vi "Main.vi"() -> ()   [LabVIEW 2018]
uses:
  TypeDefs/cntlRefs.ctl
  NistPluggableModules/BusClass/Bus.lvclass/Bus.ctl
  LV_Config_class/Typedefs/eLogLvl.ctl
  LV_Config_class/Config.lvclass/Config.ctl
  NistPluggableModules/BusClass/Accessors/Read Test.vi
  LV_Config_class/Accessors/Read ConfigFilePath.vi
  NistPluggableModules/BusClass/Accessors/Read BusNumber.vi
  <vilib>/Utility/error.llb/Error Cluster From Error Code.vi
  <vilib>/ErrorRing/Error Ring.xnode
  NistPluggableModules/TestClass/Test.lvclass
  Queue/Queue.lvlib
  <userlib>/NIST/NISTErrorLib/NISTErrorLib.lvlib
  LV_Config_class/Config.lvclass
  LV_Ini/Ini_lib.lvlib
  <vilib>/Utility/config.llb/NI_LVConfig.lvlib
  NistPluggableModules/BusClass/Bus.lvclass
  NistPluggableModules/Visualization/Visualization.lvlib
panel:
  in  "Blank Button":bool
  in  "ConfigurationList":bool[](array[boolean])
  in  "InstrumentList":u16[](array[ring]) items=["Agilent IVI FGen", "IVI Dual FGens"]
  in  "btnNHRDCPref":bool
  in  "btnNHRGSPref":bool
  in  "btnPPSPref":bool
  in  "btnChromaDCPref":bool
  in  "rngNHRDC":u16(ring) caption="NHR DC Power" items=["Agilent IVI FGen", "IVI Dual FGens"]
  in  "rngNHRG":u16(ring) caption="NHR GridSimulator" items=["Agilent IVI FGen", "IVI Dual FGens"]
  in  "rngPPS":u16(ring) caption="PPS" items=["AcPwrBase", "Chroma", "ChromaDCLoad", "NHRDCPower", "PPS"]
  in  "rngChromaDC":u16(ring) caption="ChromaDC" items=["Agilent IVI FGen", "IVI Dual FGens"]
  in  "btnChromaACPref":bool
  in  "rngChromaAC":u16(ring) caption="ChromaAC" items=["AcPwrBase", "Chroma", "ChromaDCLoad", "NHRDCPower", "PPS"]
  in  "ModuleList":string[](array[string])=["AcPwr.Chroma"]
  in  "btnRunOne":bool
  in  "btnVisualization":bool caption="Visualization"
  in  "btnHide":bool caption="Hide Modules"
  in  "btnSettings":bool
  in  "btnStop":bool
  in  "btnFGenPref":bool
  in  "rngFGen":u16(ring) caption="Function Generator" items=["Agilent IVI FGen", "IVI Dual FGens"]
  in  "rngDigitizer":u16(ring) caption="Digitizer" items=["IVI Digitizer", "Analyse Waveforms", "Debug", "Ni DaqMx Digitizer", "PMU Cal", "(obsolete)", "Simulation"]
  in  "btnDigitizerPref":bool
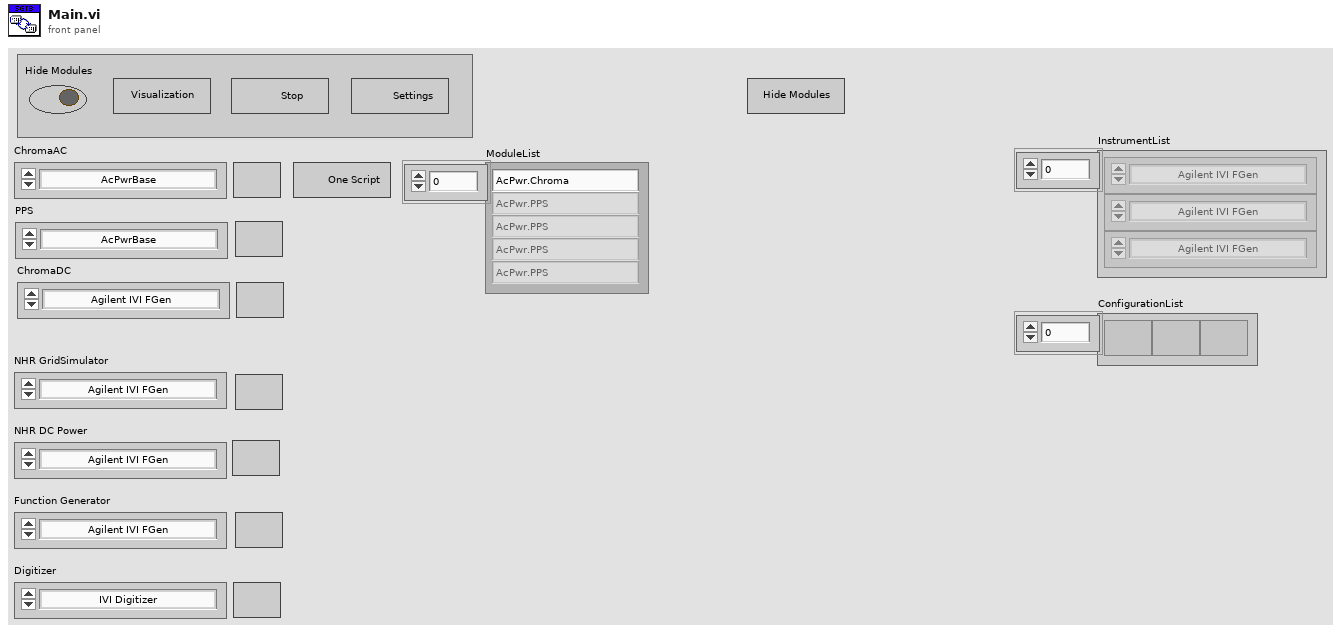
[diagram p1: front panel]
types:
  T1 = typedef "cntlRefs.ctl" = cluster{"rngFGen":refnum<vi>, "rngDigitizer":refnum<vi>, "btnHide":refnum<vi>, "rngChromaAC":refnum<vi>, "rngChromaDC":refnum<vi>, "rngPPS":refnum<vi>, "rngNHRG":refnum<vi>, "rngNHRDC":refnum<vi>}
  T2 = typedef "clUserEvents.ctl" = cluster{"StopEvent":refnum<user-event>, "RefreshUserEvents":refnum<user-event>}
  T3 = typedef "FgenModule.lvlib/clBroadcastEvents.ctl" = cluster{"DidInit":refnum<user-event>, "StatusUpdate":refnum<user-event>, "ErrorReport":refnum<user-event>, "DidStop":refnum<user-event>, "PathToINI":refnum<user-event>, "Channels":refnum<user-event>, "Function":refnum<user-event>, "Waveforms":refnum<user-event>, "Triggers":refnum<user-event>, "FunctionParams":refnum<user-event>}
  T4 = typedef "ScopeModule.lvlib/clBroadcastEvents.ctl" = cluster{"DidInit":refnum<user-event>, "StatusUpdate":refnum<user-event>, "ErrorReport":refnum<user-event>, "DidStop":refnum<user-event>, "PathToINI":refnum<user-event>, "Handle":refnum<user-event>, "Model":refnum<user-event>, "Channels":refnum<user-event>, "Acquisition":refnum<user-event>, "Trigger":refnum<user-event>, "ExtAcquisition":refnum<user-event>, "Waveform":refnum<user-event>}
  T5 = typedef "AcPwrModule.lvlib/clBroadcastEvents.ctl" = cluster{"DidInit":refnum<user-event>, "StatusUpdate":refnum<user-event>, "ErrorReport":refnum<user-event>, "DidStop":refnum<user-event>, "PathToINI":refnum<user-event>, "Measurements":refnum<user-event>, "LoadConfigFile":refnum<user-event>, "GetSettings":refnum<user-event>, "SetSettings":refnum<user-event>, "GetType&ID":refnum<user-event>}
  T6 = typedef "Config_class.lvlib/Config.lvclass/eLogLvl.ctl" = enum16{"Normal", "Verbose", "None"}
  T7 = typedef "NI_LVConfig.lvlib/Config Data RefNum.ctl" = refnum<k1>
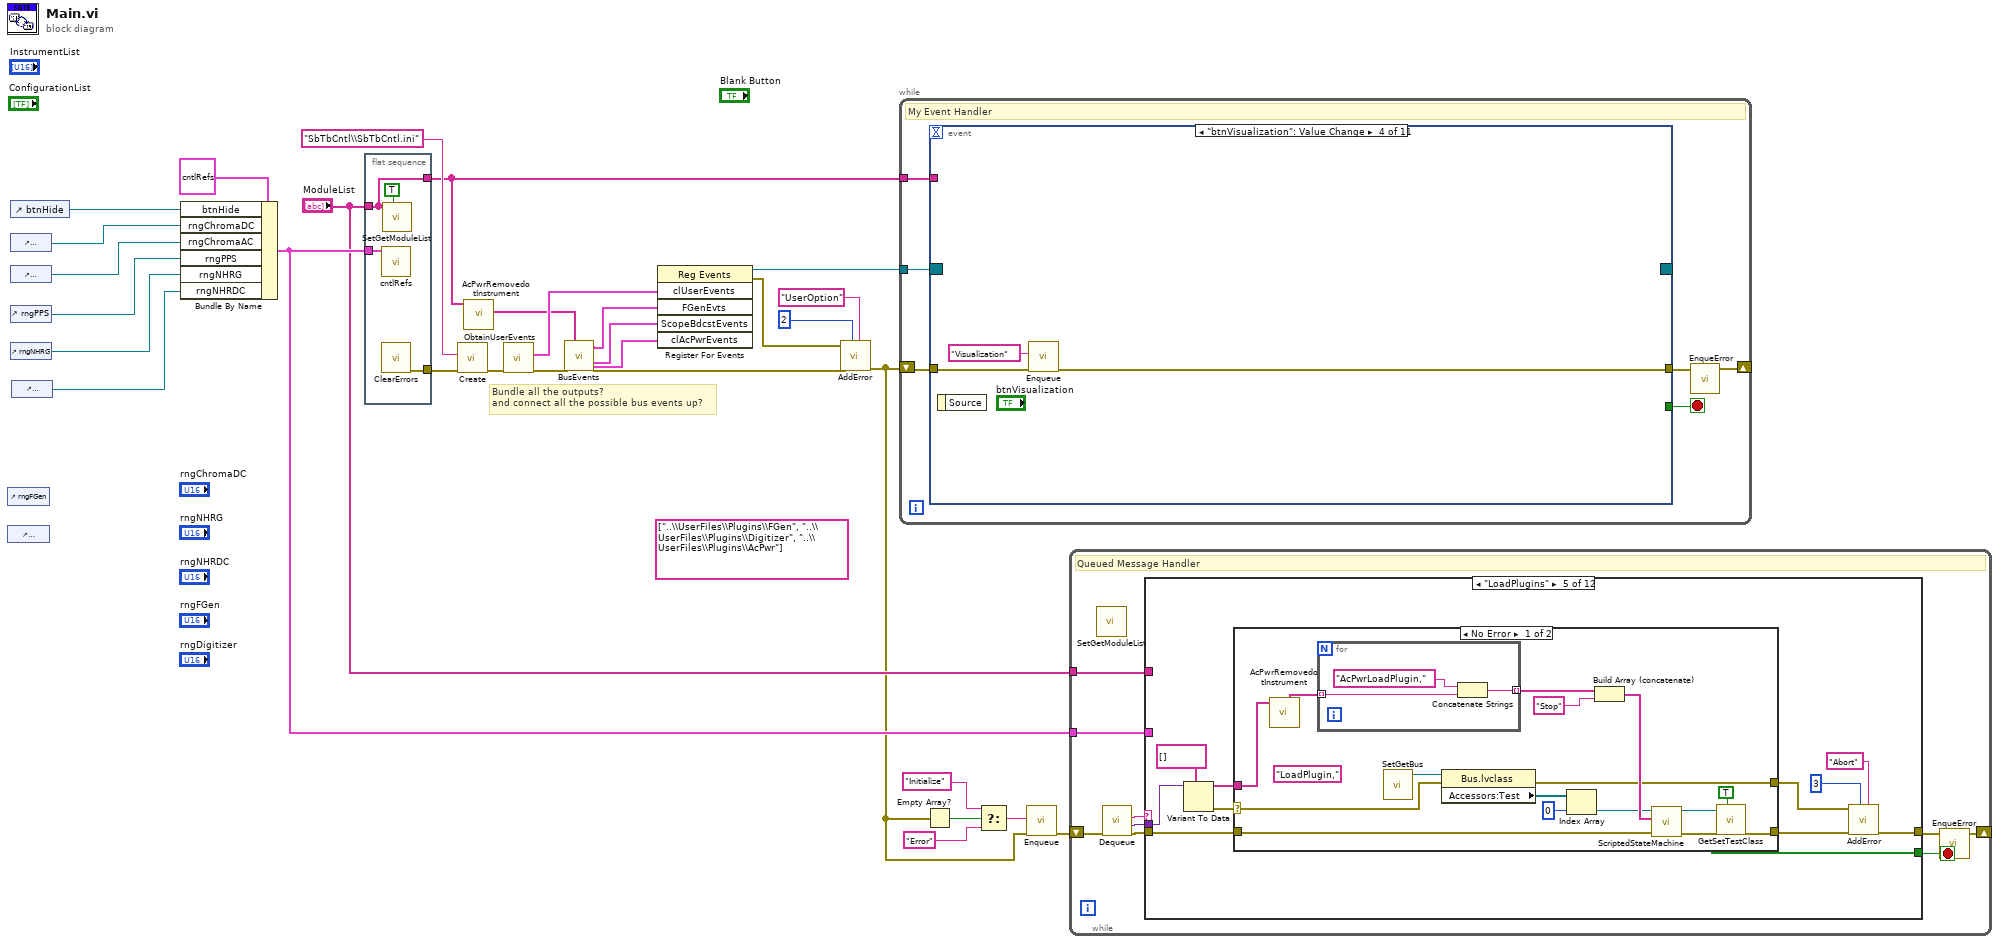
[diagram p0: block diagram]
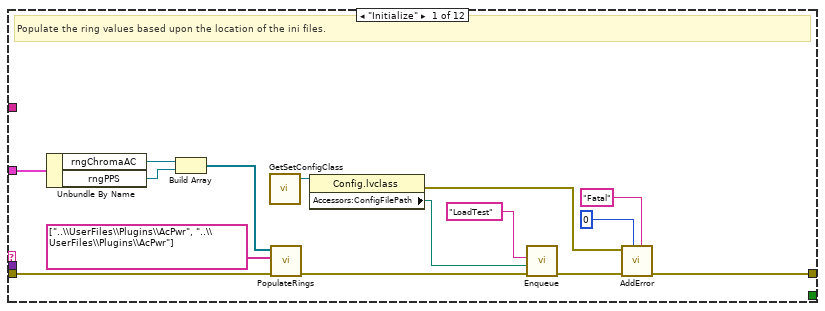
[diagram p2: hidden frame]
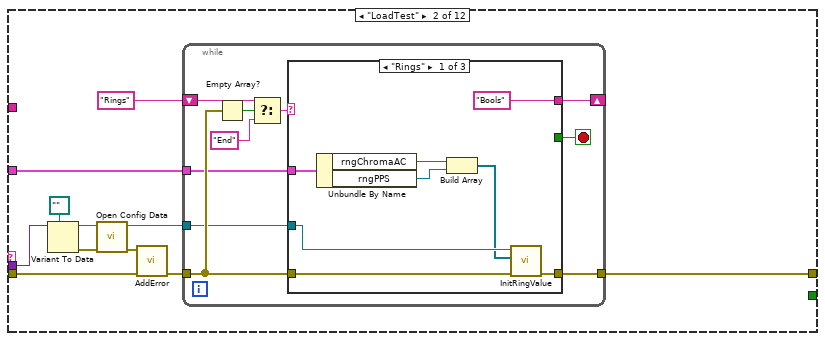
[diagram p3: hidden frame]
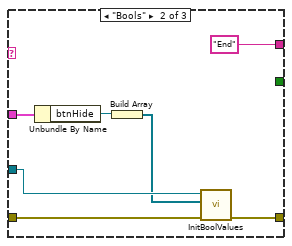
[diagram p4: hidden frame]
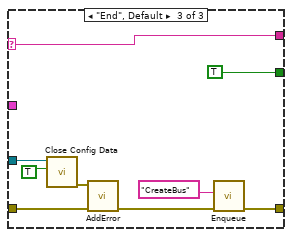
[diagram p5: hidden frame]
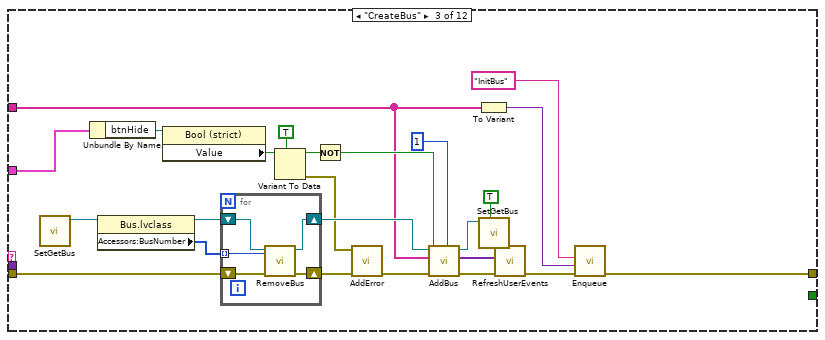
[diagram p6: hidden frame]
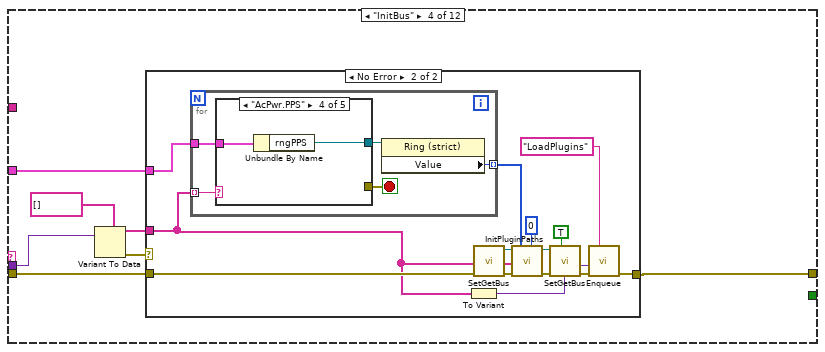
[diagram p7: hidden frame]
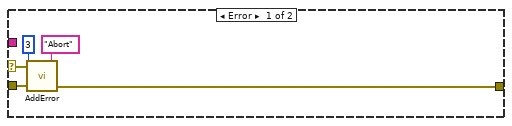
[diagram p8: hidden frame]
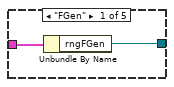
[diagram p9: hidden frame]
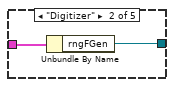
[diagram p10: hidden frame]
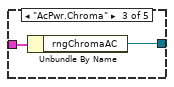
[diagram p11: hidden frame]
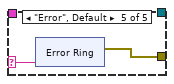
[diagram p12: hidden frame]
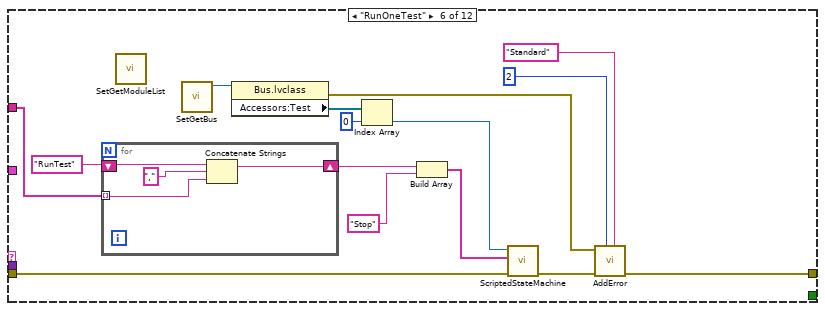
[diagram p14: hidden frame]
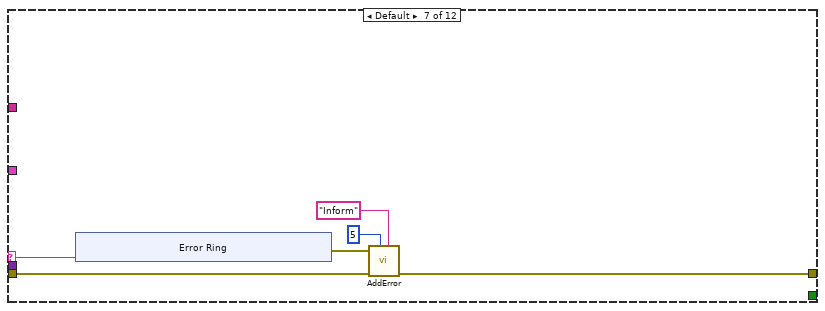
[diagram p15: hidden frame]
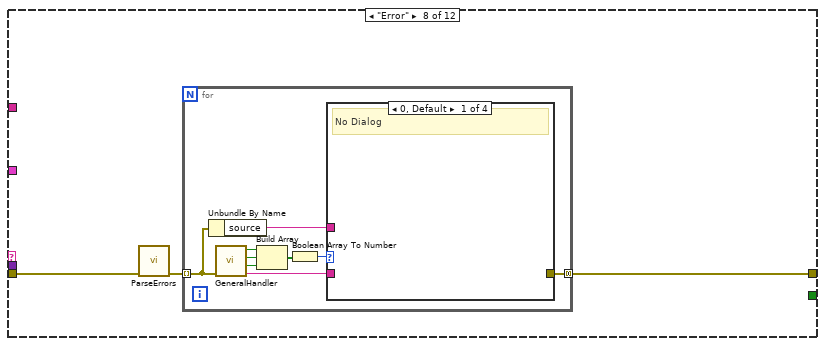
[diagram p16: hidden frame]
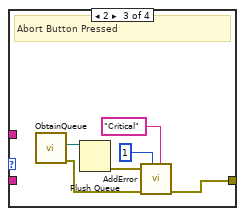
[diagram p19: hidden frame]
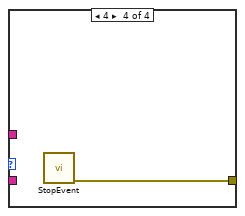
[diagram p20: hidden frame]
diagram:
  (unwired) string[] ["..\\UserFiles\\Plugins\\FGen", "..\\UserFiles\\Plugins\\Digitizer", "..\\UserFiles\\Plugins\\AcPwr"] ("RelativePathToIniArray")
  # "Bundle all the outputs? \nand connect all the possible bus events up?"
  n1 = control-ref of="rngFGen"() -> ()  [unwired: 1 out]
  n2 = control-ref of="rngDigitizer"() -> ()  [unwired: 1 out]
  n3 = control-ref of="btnHide"() -> (w15:refnum<vi>)
  n4 = control-ref of="rngChromaDC"() -> (w14:refnum<vi>)
  n5 = control-ref of="rngChromaAC"() -> (w13:refnum<vi>)
  n6 = control-ref of="rngPPS"() -> (w12:refnum<vi>)
  n7 = control-ref of="rngNHRG"() -> (w11:refnum<vi>)
  n8 = control-ref of="rngNHRDC"() -> (w10:refnum<vi>)
  n9 = Bundle By Name(cluster=T1 {"rngFGen"=refnum, "rngDigitizer"=refnum, "btnHide"=refnum, "rngChromaAC"=refnum, "rngChromaDC"=refnum, "rngPPS"=refnum, "rngNHRG"=refnum, "rngNHRDC"=refnum} ("cntlRefs"), "btnHide"=w15, "rngChromaDC"=w14, "rngChromaAC"=w13, "rngPPS"=w12, "rngNHRG"=w11, "rngNHRDC"=w10) -> (w9:T1)
  n10 = flat-sequence {
    tunnel: [w34] -> w19
    tunnel: w9 -> [w33]
    tunnel: "ModuleList" -> [w31]
    tunnel: [w31] -> w2
    frame #0 {
      n11 = call "cntlRefs.vi"("cntlRefs"=w33) -> ()  [unwired: 10 in, 1 out]
      n12 = call <userlib>:"ClearErrors.vi"() -> ("ErrorArray"=w34:errorcluster[])  [unwired: 11 in]
      n13 = call "SetGetModuleList.vi"("Set? (f)"=TRUE, "ModuleList"=w31) -> ()  [unwired: 9 in, 1 out]
    }
  }
  n14 = call "Create.vi"("ErrorArray"=w19, "name or relative path"="SbTbCntl\\SbTbCntl.ini") -> ("ErrorArray"=w20:errorcluster[])  [unwired: 8 in, 1 out]
  n15 = call "AcPwrRemovedotInstrument.vi"("ModuleList"=w2) -> ("BeforeMatch-RedundantEntries"=w1:string[])  [unwired: 8 in, 2 out]
  n16 = call "ObtainUserEvents.vi"("ErrorArray"=w20) -> ("ErrorArray"=w21:errorcluster[], "clUserEvents"=w29:T2)  [unwired: 9 in]
  n17 = call "BusEvents.vi"("Error in"=w21, "ModuleList"=w1) -> ("FGenEvts"=w16:T3, "ScopeBdcstEvents"=w18:T4, "clAcPwrEvents"=w17:T5, "Error out"=w6:errorcluster[])  [unwired: 18 in, 4 out]
  n18 = register-events(w29, w16, w18, w17) -> (reference out=w30:refnum<event-registration>, error out=w5:errorcluster)  [unwired: 2 in]
  n19 = call <userlib>:"AddError.vi"("Severity"="UserOption", "Priority"=u8 2, "ErrorArray"=w6, "error in (no error)"=w5) -> ("ErrorArray"=w3:errorcluster[])  [unwired: 6 in, 1 out]
  n20 = while {
    tunnel: w30 -> [w40]
    shift-right: [w37] -> _
    shift-left: w3 -> [w39]
    tunnel: w2 -> [w35]
    stop <- w36 stop-if-true
    # "My Event Handler"
    n21 = event shown="[3] \"btnVisualization\": Value Change" {
      selector: w40 -> [_ _ _ _ _ _ _ _ _ w210 _]
      dyn-events: [_ _ _ _ _ _ _ _ _ w211 _] -> _
      timeout: _ -> [_ _ _ _ _ _ _ _ _ _ _]
      tunnel: w39 -> [w42 w47 w61 w70 w73 w76 w123 w173 w187 w201 w214]
      tunnel: [w41 w46 w62 w69 w72 w77 w124 w164 w183 w199 w213] -> w38
      tunnel: [_ "btnStop" _ _ _ _ _ _ _ _ TRUE] -> w36
      tunnel: w35 -> [_ _ w49 _ _ _ _ _ _ w204 _]
      event "btnSettings": Value Change {
        n22 = event-data() -> ()  [unwired: 1 in, 1 out]
        n23 = call "Settings.vi"("ErrorArray"=w42) -> ("ErrorArray"=w41:errorcluster[])  [unwired: 10 in]
      }
      event "btnStop": Value Change {
        # "Stops the Framework and sends a message to the queued message handler to stop."
        n24 = event-data() -> ()  [unwired: 1 in, 1 out]
        n25 = call "Enqueue.vi"("Priority (F)"=TRUE, "ErrorArray"=w47, "Message"="Stop") -> ("ErrorArray"=w46:errorcluster[])  [unwired: 8 in]
      }
      event "btnHide": Value Change {
        # "Displays the modules need to fix this for AcPwr"
        n26 = event-data() -> ("NewVal"=w57:bool)  [unwired: 1 in]
        n27 = call "AcPwrRemovedotInstrument.vi"("ModuleList"=w49) -> ("Before Match"=w48:string[])  [unwired: 8 in, 2 out]
        n28 = call "SetGetBus.vi"() -> ("Bus.lvclass"=w60:refnum<class "Bus.lvclass">)  [unwired: 11 in]
        n29 = call "SetGetModuleList.vi"() -> ()  [unwired: 11 in, 1 out]
        n30 = property class="Bus.lvclass"(reference=w60) -> ("Accessors:Test"=w59:refnum<class "Test.lvclass">[])  [unwired: 1 in, 2 out]
        n31 = Select(t="false", s=w57, f="true") -> (s? t:f=w50:string)
        n32 = for {
          tunnel: [w67] -> w51 mode=indexing
          tunnel: w48 -> [w65] mode=indexing
          tunnel: w50 -> [w63]
          n33 = Concatenate Strings("AcPwrHideModule,", w65, ",", w63) -> (w67:string)
        }
        n34 = Index Array(array=w59, index=0) -> (element=w58:refnum<class "Test.lvclass">)
        n35 = Build Array (concatenate)(w51, "Stop") -> (w53:string[])
        n36 = call "ScriptedStateMachine.vi"("ErrorArray"=w61, "script"=w53, "Test.lvclass"=w58) -> ("ErrorArray"=w62:errorcluster[])  [unwired: 6 in, 2 out]
      }
      event "btnVisualization": Value Change {
        n37 = event-data() -> ()  [unwired: 1 in, 1 out]
        n38 = call "Enqueue.vi"("ErrorArray"=w70, "Message"="Visualization") -> ("ErrorArray"=w69:errorcluster[])  [unwired: 9 in]
      }
      event "btnRunOne": Value Change {
        # "Runs a single test?"
        n39 = event-data() -> ()  [unwired: 1 in, 1 out]
        n40 = call "Enqueue.vi"("ErrorArray"=w73, "Message"="RunOneTest") -> ("ErrorArray"=w72:errorcluster[])  [unwired: 9 in]
      }
      event "btnFGenPref", "btnDigitizerPref", "btnChromaACPref", "btnChromaDCPref", "btnPPSPref", "btnNHRGSPref", "btnNHRDCPref": Value Change {
        # "Sends a command to open up the preferences dialog. This case needs some more work but is currently runnable"
        n41 = event-data() -> ("CtlRef"=w80:refnum<vi>)  [unwired: 1 in]
        n42 = property class="Bool (strict)"(reference=w80) -> (error out=w74:errorcluster, "Label.Text"=w79:string)  [unwired: 1 in, 1 out]
        n43 = case shown="\"btnPPSPref\"" w79 {
          selector: w79 -> [_ _ _ _ w108]
          tunnel: ["Digitizer" "FGen" "Chroma" "PPS" "Error"] -> w78
          tunnel: [w98 w100 w102 w104 w107] -> w75
          tunnel: w74 -> [w98 w100 w102 w104 _]
          frame "btnDigitizerPref" {
          }
          frame "btnFGenPref" {
          }
          frame "btnChromaACPref" {
          }
          frame "btnPPSPref" {
          }
          frame Default {
            n44 = xnode "Error Ring"("parameter 0"=w108) -> ("error out"=w107:errorcluster)
          }
        }
        n45 = case shown="No Error" w75 {
          selector: w75 -> [w82 w95]
          tunnel: w78 -> [w83 _]
          tunnel: [w91 w97] -> w77
          tunnel: w76 -> [w90 w96]
          frame No Error {
            (unwired) "PrefDlgRequest," ("string")
            n46 = call "SetGetBus.vi"() -> ("Bus.lvclass"=w87:refnum<class "Bus.lvclass">)  [unwired: 11 in]
            n47 = property class="Bus.lvclass"(reference=w87, error in=w82) -> ("Accessors:Test"=w86:refnum<class "Test.lvclass">[])  [unwired: 2 out]
            n48 = Concatenate Strings("AcPwrPrefDlg," ("string"), w83) -> (w92:string)
            n49 = Build Array(w92, "Stop" ("element")) -> (w89:string[])
            n50 = Index Array(array=w86, index=0) -> (element=w85:refnum<class "Test.lvclass">)
            n51 = call "ScriptedStateMachine.vi"("ErrorArray"=w90, "script"=w89, "Test.lvclass"=w85) -> ("ErrorArray"=w91:errorcluster[])  [unwired: 6 in, 2 out]
          }
          frame Error {
            n52 = call <userlib>:"AddError.vi"("Severity"="Abort", "Priority"=u8 0, "ErrorArray"=w96, "error in (no error)"=w95) -> ("ErrorArray"=w97:errorcluster[])  [unwired: 6 in, 1 out]
          }
        }
      }
      event "rngFGen", "rngDigitizer", "rngChromaAC", "rngChromaDC", "rngPPS", "rngNHRG", "rngNHRDC": Value Change {
        # "Also needs some work"
        n53 = event-data() -> ("CtlRef"=w128:refnum<vi>)  [unwired: 1 in]
        n54 = call "SetGetBus.vi"() -> ("Bus.lvclass"=w122:refnum<class "Bus.lvclass">)  [unwired: 11 in]
        n55 = property class="Bus.lvclass"(reference=w122) -> (error out=w116:errorcluster, "Accessors:Test"=w119:refnum<class "Test.lvclass">[])  [unwired: 1 in, 1 out]
        n56 = property class="Ring (strict)"(reference=w128, error in=w116) -> (error out=w117:errorcluster, "Label.Text"=w127:string, "Value"=w121:u16)  [unwired: 1 out]
        n57 = Index Array(array=w119, index=0) -> (element=w118:refnum<class "Test.lvclass">)
        n58 = case shown="\"ChromaAC\"" w127 {
          selector: w127 -> [w146 _ _ _ _]
          tunnel: [_ "Digitizer" "FGen" "Chroma" "PPS"] -> w126
          tunnel: [w145 w152 w154 w156 w158] -> w125
          tunnel: w117 -> [_ w152 w154 w156 w158]
          frame Default {
            n59 = xnode ("Error Ring")("parameter 0"=w146) -> ("error out"=w145:errorcluster)
          }
          frame "rngDigitizer" {
          }
          frame "rngFGen" {
          }
          frame "ChromaAC" {
          }
          frame "PPS" {
          }
        }
        n60 = case shown="No Error" w125 {
          selector: w125 -> [_ w142]
          tunnel: w126 -> [w132 _]
          tunnel: [w138 w144] -> w124
          tunnel: w123 -> [w134 w143]
          tunnel: w121 -> [w133 _]
          tunnel: w118 -> [w131 _]
          frame No Error {
            (unwired) "LoadPlugin," ("string")
            n61 = call "UpdatePluginIndex.vi"("Error"=w134, "Index"=w133, "PluginName"=w132, "Test"=w131) -> ("Error"=w135:errorcluster[], "Test"=w130:refnum<class "Test.lvclass">)  [unwired: 6 in]
            n62 = Concatenate Strings("AcPwrLoadPlugin," ("string"), w132) -> (w139:string)
            n63 = Build Array(w139, "Stop") -> (w137:string[])
            n64 = call "ScriptedStateMachine.vi"("ErrorArray"=w135, "script"=w137, "Test.lvclass"=w130) -> ("ErrorArray"=w138:errorcluster[])  [unwired: 6 in, 2 out]
          }
          frame Error {
            n65 = call <userlib>:"AddError.vi"("Severity"="Abort", "Priority"=u8 3, "ErrorArray"=w143, "error in (no error)"=w142) -> ("ErrorArray"=w144:errorcluster[])  [unwired: 6 in, 1 out]
          }
        }
      }
      event User Event {
        # "Logs any error that occurs in each module"
        n66 = event-data() -> ("ModuleID"=w172:i32, "Data"=w177:variant)  [unwired: 1 in]
        n67 = Get Date/Time In Seconds() -> (seconds since 1Jan1904=w176:timestamp)
        n68 = Get Date/Time String(date format (0)=enum16{"short", "long", "abbreviated"}."short", seconds (now)=w176, want seconds? (F)=TRUE) -> (time string=w175:string)  [unwired: 1 out]
        n69 = Variant To Data(type=errorcluster {"status"=FALSE, "code"=0, "source"=""} ("error in (no error)"), Variant=w177) -> (data=w167:errorcluster, error out=w169:errorcluster)  [unwired: 1 in]
        n70 = Unbundle By Name(w167) -> ("source"=w166:string)
        n71 = Merge Errors(w167, w169) -> (w161:errorcluster)
        n72 = Format Into String(format string="%s: Module %d: %s \\r", error in=w161, w175, w172, w166) -> (resulting string=w162:string, error out=w160:errorcluster)  [unwired: 1 in]
        n73 = call <userlib>:"AddError.vi"("Severity"="Standard", "Priority"=u8 2, "ErrorArray"=w173, "error in (no error)"=w160) -> ("ErrorArray"=w165:errorcluster[])  [unwired: 6 in, 1 out]
        n74 = call "LogMessage.vi"("eLogLvl"=eLogLvl."Normal" ("LogLevel"), "Error"=w165, "LogMessage"=w162) -> ("Error"=w164:errorcluster[])  [unwired: 8 in]
      }
      event User Event {
        # "Logs and Status Update from the modules"
        n75 = event-data() -> ("Data"=w193:variant)  [unwired: 1 in]
        n76 = Get Date/Time In Seconds() -> (seconds since 1Jan1904=w194:timestamp)
        n77 = Variant To Data(type="", Variant=w193) -> (data=w190:string, error out=w192:errorcluster)  [unwired: 1 in]
        n78 = Get Date/Time String(date format (0)=enum16{"short", "long", "abbreviated"}."short", seconds (now)=w194, want seconds? (F)=TRUE) -> (time string=w191:string)  [unwired: 1 out]
        n79 = Format Into String(format string="%s: %s \\r", error in=w192, w191, w190) -> (resulting string=w180:string, error out=w186:errorcluster)  [unwired: 1 in]
        n80 = call <userlib>:"AddError.vi"("Severity"="Inform", "Priority"=u8 4, "ErrorArray"=w187, "error in (no error)"=w186) -> ("ErrorArray"=w182:errorcluster[])  [unwired: 6 in, 1 out]
        n81 = call "LogMessage.vi"("eLogLvl"=eLogLvl."Normal", "Error"=w182, "LogMessage"=w180) -> ("Error"=w183:errorcluster[])  [unwired: 8 in]
      }
      event User Event {
        # "Connect all the bus events on the external call and internal call?"
        n82 = event-data() -> ("Data"=w212:variant)  [unwired: 1 in]
        n83 = Variant To Data(type=variant[] [] ("UsrEvents"), Variant=w212) -> (data=w209:variant[], error out=w203:errorcluster)  [unwired: 1 in]
        n84 = call "SetGetModuleList.vi"() -> ()  [unwired: 11 in, 1 out]
        n85 = call "BusEvents.vi"("EventArray"=w209, "Error in"=w201, "ModuleList"=w204) -> ("FGenEvts"=w205:T3, "ScopeBdcstEvents"=w206:T4, "clAcPwrEvents"=w207:T5, "Error out"=w200:errorcluster[])  [unwired: 17 in, 4 out]
        n86 = register-events(reference=w210, error in=w203, w205, w206, w207) -> (reference out=w211:refnum<event-registration>, error out=w202:errorcluster)  [unwired: 1 in]
        n87 = call <userlib>:"AddError.vi"("Severity"="Fatal", "Priority"=u8 0, "ErrorArray"=w200, "error in (no error)"=w202) -> ("ErrorArray"=w199:errorcluster[])  [unwired: 6 in, 1 out]
      }
      event User Event {
        # "Queued Message Handler stops for any reason this top loop needs to also stop or an external stop call."
        n88 = event-data() -> ()  [unwired: 1 in, 1 out]
        n89 = call "Enqueue.vi"("Priority (F)"=TRUE, "ErrorArray"=w214, "Message"="Stop") -> ("ErrorArray"=w213:errorcluster[])  [unwired: 8 in]
      }
    }
    n90 = call "EnqueError.vi"("ErrorArrayIn"=w38) -> ("ErrorArrayOut"=w37:errorcluster[])  [unwired: 10 in]
  }
  n91 = Empty Array?(array=w3) -> (empty?=w25:bool)
  n92 = Select(t="Initialize" ("Message"), s=w25, f="Error") -> (s? t:f=w22:string)
  n93 = call "Enqueue.vi"("ErrorArray"=w3, "Message"=w22) -> ("ErrorArray"=w28:errorcluster[])  [unwired: 9 in]
  n94 = while {
    shift-right: [w223] -> _
    shift-left: w28 -> [w226]
    tunnel: w9 -> [w219]
    tunnel: "ModuleList" -> [w218]
    stop <- w221 stop-if-true
    # "Queued Message Handler"
    n95 = call "SetGetModuleList.vi"() -> ()  [unwired: 11 in, 1 out]
    n96 = call "Dequeue.vi"("ErrorArray"=w226) -> ("ErrorArray"=w222:errorcluster[], "Message Data"=w220:variant, "Message"=w225:string)  [unwired: 8 in]
    n97 = case shown="\"LoadPlugins\"" w225 {
      selector: w225 -> [_ _ _ _ _ _ w414 _ _ _ _ _]
      tunnel: [w227 w251 w300 w320 w362 w391 w413 w423 w443 w447 w466 w502] -> w224
      tunnel: w222 -> [w241 w248 w310 w321 w368 w401 w412 w422 w444 w446 w460 w506]
      tunnel: [_ _ _ _ _ _ _ _ _ _ _ TRUE] -> w221
      tunnel: w220 -> [_ w244 _ w322 w367 _ _ _ _ _ w464 _]
      tunnel: w219 -> [w234 w242 w288 w316 _ _ _ _ _ _ w456 _]
      tunnel: w218 -> [_ _ w287 _ _ w390 _ _ _ _ _ _]
      frame "Initialize" {
        # "Populate the ring values based upon the location of the ini files."
        n98 = Unbundle By Name(w234) -> ("rngChromaAC"=w233:refnum<vi>, "rngPPS"=w232:refnum<vi>)
        n99 = Build Array(w233, w232) -> (w235:refnum<vi>[])
        n100 = call "GetSetConfigClass.vi"() -> ("Ref out"=w237:refnum<class "Config.lvclass">)  [unwired: 11 in]
        n101 = call "PopulateRings.vi"("ErrorArray In"=w241, "RelativePathToIniArray"=string[] ["..\\UserFiles\\Plugins\\AcPwr", "..\\UserFiles\\Plugins\\AcPwr"], "RingRefArray"=w235) -> ("ErrorArray Out"=w239:errorcluster[])  [unwired: 7 in, 1 out]
        n102 = property class="Config.lvclass"(reference=w237) -> (error out=w229:errorcluster, "Accessors:ConfigFilePath"=w236:path)  [unwired: 1 in, 1 out]
        n103 = call "Enqueue.vi"("ErrorArray"=w239, "Message Data"=w236, "Message"="LoadTest") -> ("ErrorArray"=w228:errorcluster[])  [unwired: 8 in]
        n104 = call <userlib>:"AddError.vi"("Severity"="Fatal", "Priority"=u8 0, "ErrorArray"=w228, "error in (no error)"=w229) -> ("ErrorArray"=w227:errorcluster[])  [unwired: 6 in, 1 out]
      }
      frame "LoadTest" {
        n105 = Variant To Data(type=path "", Variant=w244) -> (data=w245:path, error out=w250:errorcluster)  [unwired: 1 in]
        n106 = call <vilib>:"Open Config Data.vi"("error in (no error)"=w250, "configuration file path"=w245) -> ("error out"=w247:errorcluster, "refnum"=w243:T7)  [unwired: 7 in, 1 out]
        n107 = call <userlib>:"AddError.vi"("ErrorArray"=w248, "error in (no error)"=w247) -> ("ErrorArray"=w249:errorcluster[])  [unwired: 8 in, 1 out]
        n108 = while {
          shift-right: [w262] -> _
          shift-left: "Rings" -> [w255]
          tunnel: w249 -> [w257]
          tunnel: [w259] -> w251
          tunnel: w243 -> [w254]
          tunnel: w242 -> [w253]
          stop <- w258 stop-if-true
          n109 = Empty Array?(array=w257) -> (empty?=w256:bool)
          n110 = Select(t=w255, s=w256, f="End") -> (s? t:f=w261:string)
          n111 = case shown="\"Rings\"" w261 {
            selector: w261 -> [_ _ w286]
            tunnel: ["Bools" "End" w286] -> w262
            tunnel: w257 -> [w268 w275 w281]
            tunnel: [w269 w276 w280] -> w259
            tunnel: [_ _ TRUE] -> w258
            tunnel: w254 -> [w267 w273 w284]
            tunnel: w253 -> [w265 w272 _]
            frame "Rings" {
              n112 = Unbundle By Name(w265) -> ("rngChromaAC"=w266:refnum<vi>, "rngPPS"=w264:refnum<vi>)
              n113 = Build Array(w266, w264) -> (w263:refnum<vi>[])
              n114 = call "InitRingValue.vi"("ErrorArray In"=w268, "RingRefArray"=w263, "IniFileRef"=w267) -> ("ErrorArray Out"=w269:errorcluster[])  [unwired: 6 in, 2 out]
            }
            frame "Bools" {
              n115 = Unbundle By Name(w272) -> ("btnHide"=w274:refnum<vi>)
              n116 = Build Array(w274) -> (w271:refnum<vi>[])
              n117 = call "InitBoolValues.vi"("ErrorArray in"=w275, "BoolRefArray"=w271, "IniFileRef in"=w273) -> ("ErrorArray Out"=w276:errorcluster[])  [unwired: 7 in, 1 out]
            }
            frame "End", Default {
              n118 = call <vilib>:"Close Config Data.vi"("write file if changed (T)"=TRUE, "refnum"=w284) -> ("error out"=w282:errorcluster)  [unwired: 8 in, 1 out]
              n119 = call <userlib>:"AddError.vi"("ErrorArray"=w281, "error in (no error)"=w282) -> ("ErrorArray"=w279:errorcluster[])  [unwired: 8 in, 1 out]
              n120 = call "Enqueue.vi"("ErrorArray"=w279, "Message"="CreateBus") -> ("ErrorArray"=w280:errorcluster[])  [unwired: 9 in]
            }
          }
        }
      }
      frame "CreateBus" {
        n121 = call "SetGetBus.vi"() -> ("Bus.lvclass"=w306:refnum<class "Bus.lvclass">)  [unwired: 11 in]
        n122 = Unbundle By Name(w288) -> ("btnHide"=w289:refnum<vi>)
        n123 = property class="Bus.lvclass"(reference=w306) -> (reference out=w309:refnum<class "Bus.lvclass">, "Accessors:BusNumber"=w303:i32[])  [unwired: 1 in, 1 out]
        n124 = property class="Bool (strict)"(reference=w289) -> ("Value"=w296:bool)  [unwired: 1 in, 2 out]
        n125 = for {
          shift-right: [w314] -> w292
          shift-left: w310 -> [w315]
          shift-right: [w311] -> w308
          shift-left: w309 -> [w313]
          tunnel: w303 -> [w312] mode=indexing
          n126 = call "RemoveBus.vi"("BusNumber"=w312, "ErrorIn"=w315, "Bus.lvclass"=w313) -> ("ErrorOut"=w314:errorcluster[], "Bus.lvclass"=w311:refnum<class "Bus.lvclass">)  [unwired: 7 in]
        }
        n127 = Variant To Data(type=TRUE, Variant=w296) -> (data=w295:bool, error out=w290:errorcluster)  [unwired: 1 in]
        n128 = Not(x=w295) -> (.not. x?=w293:bool)
        n129 = call <userlib>:"AddError.vi"("ErrorArray"=w292, "error in (no error)"=w290) -> ("ErrorArray"=w291:errorcluster[])  [unwired: 8 in, 1 out]
        n130 = call "AddBus.vi"("ShowPanel? (f)"=w293, "BusNumber"=1, "ErrorIn"=w291, "ModuleList"=w287, "Bus.lvclass"=w308) -> ("ErrorOut"=w302:errorcluster[], "UsrEvents"=w301:variant[], "Bus.lvclass"=w305:refnum<class "Bus.lvclass">)  [unwired: 4 in]
        n131 = To Variant(anything=w287) -> (Variant=w297:variant)
        n132 = call "SetGetBus.vi"("Set (f)"=TRUE, "Bus.lvclass"=w305) -> ()  [unwired: 9 in, 1 out]
        n133 = call "RefreshUserEvents.vi"("ErrorIn"=w302, "Data"=w301) -> ("ErrorOut"=w299:errorcluster[])  [unwired: 9 in]
        n134 = call "Enqueue.vi"("ErrorArray"=w299, "Message Data"=w297, "Message"="InitBus") -> ("ErrorArray"=w300:errorcluster[])  [unwired: 8 in]
      }
      frame "InitBus" {
        n135 = Variant To Data(type=string[] [] ("ModuleList"), Variant=w322) -> (data=w318:string[], error out=w319:errorcluster)  [unwired: 1 in]
        n136 = case shown="No Error" w319 {
          selector: w319 -> [w323 _]
          tunnel: w321 -> [w324 w335]
          tunnel: [w325 w333] -> w320
          tunnel: w318 -> [_ w329]
          tunnel: w316 -> [_ w328]
          frame Error {
            n137 = call <userlib>:"AddError.vi"("Severity"="Abort", "Priority"=u8 3, "ErrorArray"=w324, "error in (no error)"=w323) -> ("ErrorArray"=w325:errorcluster[])  [unwired: 6 in, 1 out]
          }
          frame No Error {
            n138 = for {
              tunnel: w329 -> [w343] mode=indexing
              tunnel: [w344] -> w339 mode=indexing
              tunnel: w328 -> [w340]
              stop <- w342 stop-if-true
              n139 = case shown="\"AcPwr.PPS\"" w343 {
                selector: w343 -> [_ _ _ _ w354]
                tunnel: [w346 w348 w350 w352 _] -> w341
                tunnel: [_ _ _ _ w353] -> w342
                tunnel: w340 -> [w345 w347 w349 w351 _]
                frame "FGen" {
                  n140 = Unbundle By Name(w345) -> ("rngFGen"=w346:refnum<vi>)
                }
                frame "Digitizer" {
                  n141 = Unbundle By Name(w347) -> ("rngFGen"=w348:refnum<vi>)
                }
                frame "AcPwr.Chroma" {
                  n142 = Unbundle By Name(w349) -> ("rngChromaAC"=w350:refnum<vi>)
                }
                frame "AcPwr.PPS" {
                  n143 = Unbundle By Name(w351) -> ("rngPPS"=w352:refnum<vi>)
                }
                frame "Error", Default {
                  n144 = xnode "Error Ring"("parameter 0"=w354) -> ("error out"=w353:errorcluster)
                }
              }
              n145 = property class="Ring (strict)"(reference=w341) -> ("Value"=w344:u16)  [unwired: 1 in, 2 out]
            }
            n146 = To Variant(anything=w329) -> (Variant=w330:variant)
            n147 = call "SetGetBus.vi"() -> ("Bus.lvclass"=w337:refnum<class "Bus.lvclass">)  [unwired: 11 in]
            n148 = call "InitPluginPaths.vi"("BusIndex"=0, "PluginIndex"=w339, "Error In"=w335, "Modules"=w329, "Bus in"=w337) -> ("Error Out"=w332:errorcluster[], "Bus out"=w336:refnum<class "Bus.lvclass">)  [unwired: 5 in]
            n149 = call "SetGetBus.vi"("Set (f)"=TRUE, "Bus.lvclass"=w336) -> ()  [unwired: 9 in, 1 out]
            n150 = call "Enqueue.vi"("ErrorArray"=w332, "Message Data"=w330, "Message"="LoadPlugins") -> ("ErrorArray"=w333:errorcluster[])  [unwired: 8 in]
          }
        }
      }
      frame "LoadPlugins" {
        n151 = Variant To Data(type=string[] [] ("ModuleList"), Variant=w367) -> (data=w365:string[], error out=w369:errorcluster)  [unwired: 1 in]
        n152 = case shown="No Error" w369 {
          selector: w369 -> [w374 w388]
          tunnel: w368 -> [w377 w389]
          tunnel: [w376 w389] -> w361
          tunnel: w365 -> [w373 _]
          tunnel: [w375 w388] -> w360
          frame No Error {
            (unwired) "LoadPlugin," ("string")
            n153 = call "AcPwrRemovedotInstrument.vi"("ModuleList"=w373) -> ("AfterMatch"=w372:string[])  [unwired: 8 in, 2 out]
            n154 = for {
              tunnel: [w387] -> w383 mode=indexing
              tunnel: w372 -> [w385] mode=indexing
              n155 = Concatenate Strings("AcPwrLoadPlugin," ("string"), w385) -> (w387:string)
            }
            n156 = call "SetGetBus.vi"() -> ("Bus.lvclass"=w384:refnum<class "Bus.lvclass">)  [unwired: 11 in]
            n157 = property class="Bus.lvclass"(reference=w384, error in=w374) -> (error out=w375:errorcluster, "Accessors:Test"=w381:refnum<class "Test.lvclass">[])  [unwired: 1 out]
            n158 = Index Array(array=w381, index=0) -> (element=w378:refnum<class "Test.lvclass">)
            n159 = Build Array (concatenate)(w383, "Stop") -> (w379:string[])
            n160 = call "ScriptedStateMachine.vi"("ErrorArray"=w377, "script"=w379, "Test.lvclass"=w378) -> ("ErrorArray"=w376:errorcluster[], "Test.lvclass"=w370:refnum<class "Test.lvclass">)  [unwired: 6 in, 1 out]
            n161 = call "GetSetTestClass.vi"("Set"=TRUE, "Test.lvclass"=w370) -> ()  [unwired: 9 in, 1 out]
          }
          frame Error {
          }
        }
        n162 = call <userlib>:"AddError.vi"("Severity"="Abort", "Priority"=u8 3, "ErrorArray"=w361, "error in (no error)"=w360) -> ("ErrorArray"=w362:errorcluster[])  [unwired: 6 in, 1 out]
      }
      frame "RunOneTest" {
        n163 = for {
          shift-right: [w407] -> w396
          shift-left: "RunTest" ("string") -> [w408]
          tunnel: w390 -> [w405] mode=indexing
          n164 = Concatenate Strings(w408, "," ("string"), w405) -> (w407:string)
        }
        n165 = call "SetGetModuleList.vi"() -> ()  [unwired: 11 in, 1 out]
        n166 = call "SetGetBus.vi"() -> ("Bus.lvclass"=w404:refnum<class "Bus.lvclass">)  [unwired: 11 in]
        n167 = property class="Bus.lvclass"(reference=w404) -> (error out=w393:errorcluster, "Accessors:Test"=w403:refnum<class "Test.lvclass">[])  [unwired: 1 in, 1 out]
        n168 = Index Array(array=w403, index=0) -> (element=w400:refnum<class "Test.lvclass">)
        n169 = Build Array(w396, "Stop") -> (w397:string[])
        n170 = call "ScriptedStateMachine.vi"("ErrorArray"=w401, "script"=w397, "Test.lvclass"=w400) -> ("ErrorArray"=w392:errorcluster[])  [unwired: 6 in, 2 out]
        n171 = call <userlib>:"AddError.vi"("Severity"="Standard", "Priority"=u8 2, "ErrorArray"=w392, "error in (no error)"=w393) -> ("ErrorArray"=w391:errorcluster[])  [unwired: 6 in, 1 out]
      }
      frame Default {
        n172 = xnode "Error Ring"("parameter 0"=w414) -> ("error out"=w409:errorcluster)
        n173 = call <userlib>:"AddError.vi"("Severity"="Inform", "Priority"=u8 5, "ErrorArray"=w412, "error in (no error)"=w409) -> ("ErrorArray"=w413:errorcluster[])  [unwired: 6 in, 1 out]
      }
      frame "Error" {
        n174 = call <userlib>:"ParseErrors.vi"("ErrorArray"=w422) -> ("ErrorArray"=w424:errorcluster[])  [unwired: 8 in, 2 out]
        n175 = for {
          tunnel: w424 -> [w433] mode=indexing
          tunnel: [w425] -> w423 mode=concatenating
          n176 = Unbundle By Name(w433) -> ("source"=w427:string)
          n177 = call <userlib>:"GeneralHandler.vi"("error in (no error)"=w433) -> ("Severity"=w426:string, "Stop"=w430:bool, "Abort"=w431:bool, "Continue"=w432:bool)  [unwired: 7 in]
          n178 = Build Array(w432, w431, w430) -> (w429:bool[])
          n179 = Boolean Array To Number(Boolean array=w429) -> (number=w428:u32)
          n180 = case shown="0, Default" w428 {
            tunnel: w427 -> [_ _ _ _]
            tunnel: w426 -> [_ w434 _ _]
            tunnel: [_ _ w435 w441] -> w425
            frame 0, Default {
              # "No Dialog"
            }
            frame 1 {
              # "Continue"
              n181 = case shown="Default" w434 {
                frame Default {
                  # "Continue operation"
                }
                frame "Log" {
                  # "TODO: if your program\nhas a log file.  Write to \nit here."
                  # "Write to log file"
                }
              }
            }
            frame 2 {
              # "Abort Button Pressed"
              n182 = call "ObtainQueue.vi"() -> ("ErrorArray"=w438:errorcluster[], "QueueRef"=w440:refnum<queue>)  [unwired: 10 in]
              n183 = Flush Queue(queue=w440) -> (error out=w439:errorcluster)  [unwired: 1 in, 2 out]
              n184 = call <userlib>:"AddError.vi"("Severity"="Critical", "Priority"=u8 1, "ErrorArray"=w438, "error in (no error)"=w439) -> ("ErrorArray"=w435:errorcluster[])  [unwired: 6 in, 1 out]
            }
            frame 4 {
              n185 = call "StopEvent.vi"() -> ("ErrorArray"=w441:errorcluster[])  [unwired: 11 in]
            }
          }
        }
      }
      frame "Visualization" {
        n186 = call "dlgSelectVisApps.vi"("Error In"=w444, "PathsToVisApps"=string[] ["VisualizeStatus", "VisualizeAcPwr"]) -> ("Error Out"=w443:errorcluster[])  [unwired: 9 in]
      }
      frame "Stop" {
        n187 = call "GetSetConfigClass.vi"() -> ("Ref out"=w455:refnum<class "Config.lvclass">)  [unwired: 11 in]
        n188 = property class="Config.lvclass"(reference=w455) -> (error out=w445:errorcluster, "Accessors:ConfigFilePath"=w451:path)  [unwired: 1 in, 1 out]
        n189 = call "Enqueue.vi"("ErrorArray"=w446, "Message Data"=w451, "Message"="SaveTest") -> ("ErrorArray"=w452:errorcluster[])  [unwired: 8 in]
        n190 = call "Enqueue.vi"("ErrorArray"=w452, "Message"="End") -> ("ErrorArray"=w448:errorcluster[])  [unwired: 9 in]
        n191 = call <userlib>:"AddError.vi"("Severity"="Fatal", "Priority"=u8 0, "ErrorArray"=w448, "error in (no error)"=w445) -> ("ErrorArray"=w447:errorcluster[])  [unwired: 6 in, 1 out]
      }
      frame "SaveTest" {
        n192 = Variant To Data(type=path "", Variant=w464) -> (data=w459:path, error out=w463:errorcluster)  [unwired: 1 in]
        n193 = call <vilib>:"Open Config Data.vi"("error in (no error)"=w463, "configuration file path"=w459) -> ("error out"=w462:errorcluster, "refnum"=w458:T7)  [unwired: 7 in, 1 out]
        n194 = call <userlib>:"AddError.vi"("ErrorArray"=w460, "error in (no error)"=w462) -> ("ErrorArray"=w461:errorcluster[])  [unwired: 8 in, 1 out]
        n195 = while {
          tunnel: w461 -> [w472]
          tunnel: [w476] -> w466
          shift-right: [w475] -> _
          shift-left: "Rings" -> [w473]
          tunnel: w458 -> [w468]
          tunnel: w456 -> [w467]
          stop <- w469 stop-if-true
          n196 = Empty Array?(array=w472) -> (empty?=w471:bool)
          n197 = Select(t=w473, s=w471, f="End") -> (s? t:f=w474:string)
          n198 = case shown="\"End\", Default" w474 {
            selector: w474 -> [_ _ w498]
            tunnel: w472 -> [w482 w489 w495]
            tunnel: [w481 w490 w492] -> w476
            tunnel: ["Bools" "End" w498] -> w475
            tunnel: [_ _ TRUE] -> w469
            tunnel: w468 -> [w480 w488 w494]
            tunnel: w467 -> [w479 w486 _]
            frame "Rings" {
              n199 = Unbundle By Name(w479) -> ("rngChromaAC"=w483:refnum<vi>, "rngPPS"=w478:refnum<vi>)
              n200 = Build Array(w483, w478) -> (w477:refnum<vi>[])
              n201 = call "RingsToIni.vi"("ErrorArray in"=w482, "RingRefArray"=w477, "IniFileRef in"=w480) -> ("ErrorArray out"=w481:errorcluster[])  [unwired: 7 in, 1 out]
            }
            frame "Bools" {
              n202 = Unbundle By Name(w486) -> ("btnHide"=w487:refnum<vi>)
              n203 = Build Array(w487) -> (w485:refnum<vi>[])
              n204 = call "BoolsToIni.vi"("ErrorArray in"=w489, "BoolRefArray"=w485, "IniFileRef in"=w488) -> ("ErrorArray out"=w490:errorcluster[])  [unwired: 7 in, 1 out]
            }
            frame "End", Default {
              n205 = call <vilib>:"Close Config Data.vi"("write file if changed (T)"=TRUE, "refnum"=w494) -> ("error out"=w496:errorcluster)  [unwired: 8 in, 1 out]
              n206 = call <userlib>:"AddError.vi"("ErrorArray"=w495, "error in (no error)"=w496) -> ("ErrorArray"=w492:errorcluster[])  [unwired: 8 in, 1 out]
            }
          }
        }
      }
      frame "End" {
        n207 = call "SetGetBus.vi"() -> ("Bus.lvclass"=w505:refnum<class "Bus.lvclass">)  [unwired: 11 in]
        n208 = property class="Bus.lvclass"(reference=w505) -> (reference out=w504:refnum<class "Bus.lvclass">, "Accessors:BusNumber"=w503:i32[])  [unwired: 1 in, 1 out]
        n209 = for {
          tunnel: w503 -> [w509] mode=indexing
          shift-right: [w511] -> w502
          shift-left: w506 -> [w508]
          shift-right: [w507] -> w501
          shift-left: w504 -> [w510]
          n210 = call "RemoveBus.vi"("BusNumber"=w509, "ErrorIn"=w508, "Bus.lvclass"=w510) -> ("ErrorOut"=w511:errorcluster[], "Bus.lvclass"=w507:refnum<class "Bus.lvclass">)  [unwired: 7 in]
        }
        n211 = call "SetGetBus.vi"("Set (f)"=TRUE, "Bus.lvclass"=w501) -> ()  [unwired: 9 in, 1 out]
      }
    }
    n212 = call "EnqueError.vi"("ErrorArrayIn"=w224) -> ("ErrorArrayOut"=w223:errorcluster[])  [unwired: 10 in]
  }
